vi "Motor with Encoder - DrH Test v2.vi"() -> ()   [LabVIEW 2016]
doc: "This example shows how to move a motor connected to an encoder and a wheel, and then read information about the system from an encoder.\n\nThis is an example of how to use feedback (from the encoder) to create an open loop system. If some control method was used, for example using PID, a closed loop system could be created.\n\nThis example expects a USB cable connected from your development PC to the Type B USB Jack (next to the power input) on the roboRIO.\n\nThis example requires the Driver Station to be running with Teleoperated Enabled."
uses:
  <vilib>/Rock Robotics/SystemInterfaces/DIO/FPGA_DIOChannel.ctl
  <vilib>/Rock Robotics/WPI/Encoder/WPI_EncoderType.ctl
  <vilib>/Rock Robotics/SystemInterfaces/DIO/FPGA_DIOPWMChannel.ctl
  <vilib>/Rock Robotics/WPI/Counter/WPI_CounterDigitalInputToDigitalSource.vi
  <vilib>/Rock Robotics/WPI/MotorControl/WPI_MotorControlOpen SPARK.vi
panel:
  out "Encoder Rate (RPM) 2":dbl
  out "XY Graph":cluster{dbl[], dbl[]}(graph)
  out "Waveform Chart":dbl(graph)
  in  "Motor Speed (-1 to 1)":dbl(slide) scale=-1.0..1.0
  in  "Motor PWM Channel":T1=enum."PWM 9"
  in  "Number Samples to Average":u8=1 min=1 max=128
  in  "Invert Direction":bool
  in  "Decoding Type":T2=enum."4x"
  in  "DistancePerCount (deg)":dbl=0.351563
  in  "Encoder B Channel":T3=enum."DIO 1"
  in  "Encoder A Channel":T3
  out "Encoder Rate (deg/sec)":dbl
  in  "Minimum Rate":dbl=20.0
  in  "Stop":bool
  out "Encoder Alarm Status":string="Encoder Stopped"
  out "Encoder Direction":string="Forward"
  # "These can be set while running."
  # "Output information."
  # "Set these inputs before running."
  # "This example requires the Driver Station to be running with Teleoperated Enabled."
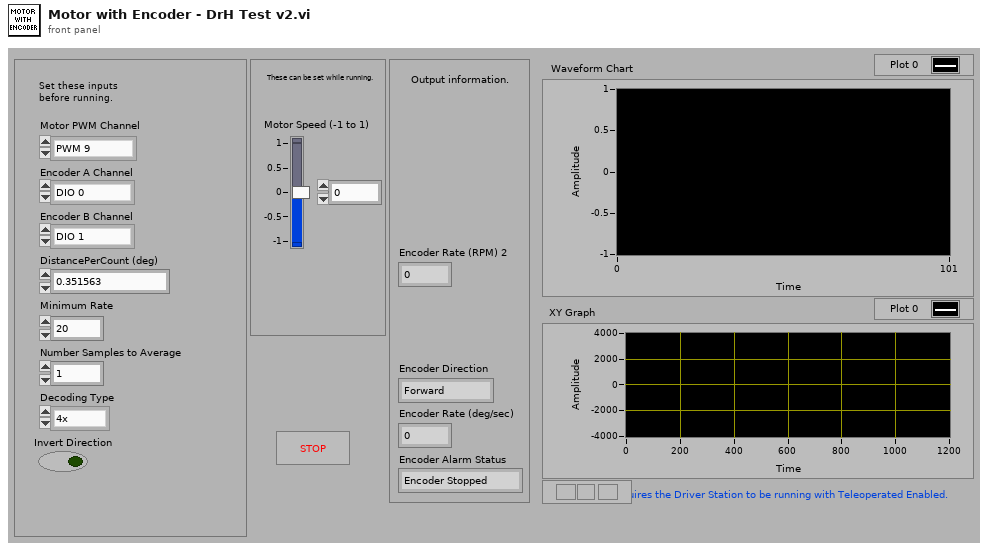
[diagram p1: front panel]
types:
  T1 = typedef "FPGA_DIOPWMChannel.ctl" = enum8{"PWM 0", "PWM 1", "PWM 2", "PWM 3", "PWM 4", "PWM 5", "PWM 6", "PWM 7", "PWM 8", "PWM 9", "PWM MXP 0", "PWM MXP 1", "PWM MXP 2", "PWM MXP 3", "PWM MXP 4", "PWM MXP 5", "PWM MXP 6", "PWM MXP 7", "PWM MXP 8", "PWM MXP 9", "Invalid"}
  T2 = typedef "WPI_EncoderType.ctl" = enum16{"1x", "2x", "4x"}
  T3 = typedef "FPGA_DIOChannel.ctl" = enum8{"DIO 0", "DIO 1", "DIO 2", "DIO 3", "DIO 4", "DIO 5", "DIO 6", "DIO 7", "DIO 8", "DIO 9", "DIO MXP 0", "DIO MXP 1", "DIO MXP 2", "DIO MXP 3", "DIO MXP 4", "DIO MXP 5", "DIO MXP 6", "DIO MXP 7", "DIO MXP 8", "DIO MXP 9", "DIO MXP 10", "DIO MXP 11", "DIO MXP 12", "DIO MXP 13", "DIO MXP 14", "DIO MXP 15", "SPI Port CS1", "SPI Port CS2", "SPI Port CS3", "SPI Port MISO", "SPI Port MOSI", "Invalid"}
  T4 = typedef "WPI_MotorControlDeviceRef.ctl" = cluster{"DeviceStatus":errorcluster, "Type":T5, "PWM":cluster{"PWM Channel":T1, "DeadBand":T6}, "CAN":cluster{"Device Number":u8, "SetOutput VI Ref":variant, "GetOutput VI Ref":variant, "Enable VI Ref":variant, "Disable VI Ref":variant, "Data":variant}, "Invert":bool}
  T5 = typedef "WPI_MotorControlType.ctl" = enum16{"PWM", "CAN"}
  T6 = typedef "WPI_PWMDeadband.ctl" = cluster{"Name":string, "maxPositivePwm":i32, "minPositivePwm":i32, "centerPwm":i32, "maxNegativePwm":i32, "minNegativePwm":i32, "angularRange":u16}
  T7 = typedef "WPI_DigitalInputDevRef.ctl" = cluster{"DevStatus":errorcluster, "DIO Channel":T3}
  T8 = typedef "FPGA_CounterEncoderSourceConvertionLVSourceType.ctl" = cluster{"DevStatus":errorcluster, "AnalogTriggerMode?":bool, "DigitalMode":cluster{"DIO Channel":T9}, "AnalogTriggerMode":cluster{"AnalogTriggerIndex":T10, "OutputType":T11}}
  T9 = typedef "FPGA_DIODigitalSourceChannel.ctl" = enum8{"DIO 0", "DIO 1", "DIO 2", "DIO 3", "DIO 4", "DIO 5", "DIO 6", "DIO 7", "DIO 8", "DIO 9", "DIO MXP 0", "DIO MXP 1", "DIO MXP 2", "DIO MXP 3", "DIO MXP 4", "DIO MXP 5", "DIO MXP 6", "DIO MXP 7", "DIO MXP 8", "DIO MXP 9", "DIO MXP 10", "DIO MXP 11", "DIO MXP 12", "DIO MXP 13", "DIO MXP 14", "DIO MXP 15", "Disabled"}
  T10 = typedef "FPGA_AnalogTriggerIndex.ctl" = enum8{"Trig 0", "Trig 1", "Trig 2", "Trig 3", "Trig 4", "Trig 5", "Trig 6", "Trig 7", "Invalid"}
  T11 = typedef "FPGA_AnalogTriggerOutType.ctl" = enum16{"InWindow", "TriggerState", "Rising", "Falling"}
  T12 = typedef "WPI_EncoderDevRef.ctl" = cluster{"DevStatus":errorcluster, "EncoderIndex":T13, "CounterIndex":T14, "DistancePerCount":dbl, "Decoding Type":T2}
  T13 = typedef "FPGA_EncoderIdx.ctl" = enum8{"Enc 0", "Enc 1", "Enc 2", "Enc 3", "Enc 4", "Enc 5", "Enc 6", "Enc 7", "Invalid"}
  T14 = typedef "FPGA_CounterCtrSystemIndex.ctl" = enum8{"Ctr 0", "Ctr 1", "Ctr 2", "Ctr 3", "Ctr 4", "Ctr 5", "Ctr 6", "Ctr 7", "Invalid"}
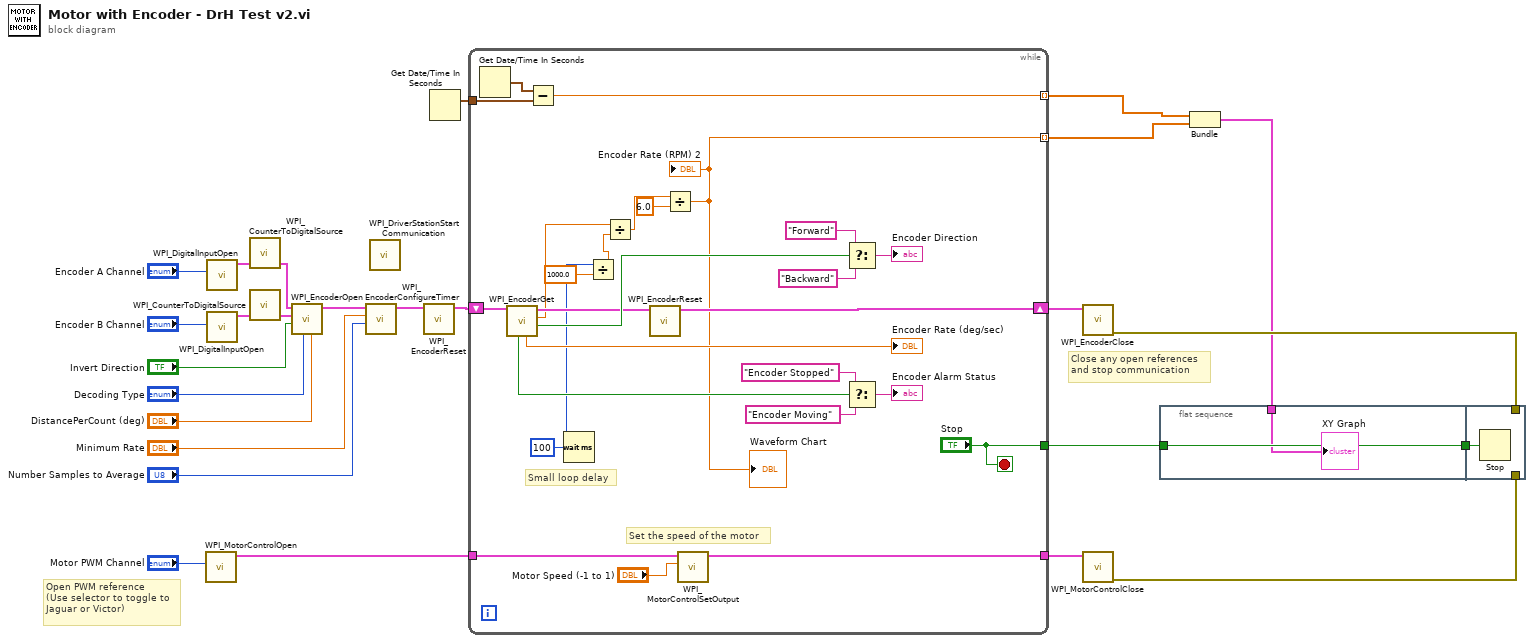
[diagram p0: block diagram]
diagram:
  # "Open PWM reference\n(Use selector to toggle to Jaguar or Victor)"
  # "Close any open references\nand stop communication"
  n1 = call-poly <vilib>:"WPI_MotorControlOpen.vi"("PWM Channel"="Motor PWM Channel") -> ("MotorControlDeviceRef"=w12:T4)  [unwired: 3 in, 7 out]
  n2 = call <vilib>:"WPI_DigitalInputOpen.vi"("DIO Channel"="Encoder A Channel") -> ("DigitalInputDevRef"=w23:T7)  [unwired: 1 in, 9 out]
  n3 = call <vilib>:"WPI_DigitalInputOpen.vi"("DIO Channel"="Encoder B Channel") -> ("DigitalInputDevRef"=w24:T7)  [unwired: 1 in, 9 out]
  n4 = call-poly <vilib>:"WPI_CounterToDigitalSource.vi"("DigitalInputDevRef"=w23) -> ("Digital Source"=w22:T8)  [unwired: 6 out]
  n5 = call-poly <vilib>:"WPI_CounterToDigitalSource.vi"("DigitalInputDevRef"=w24) -> ("Digital Source"=w25:T8)  [unwired: 6 out]
  n6 = call <vilib>:"WPI_EncoderOpen.vi"("DistancePerCount"="DistancePerCount (deg)", "Decoding Type"="Decoding Type", "Invert Direction (False)"="Invert Direction", "BSource"=w25, "ASource"=w22) -> ("EncoderDevRef"=w16:T12)  [unwired: 3 in, 3 out]
  n7 = call <vilib>:"WPI_EncoderConfigureTimer.vi"("Number Samples to Average"="Number Samples to Average", "Minimum Rate"="Minimum Rate", "EncoderDevRef"=w16) -> ("EncoderDevRef"=w4:T12)  [unwired: 1 in, 7 out]
  n8 = call <vilib>:"WPI_DriverStationStart Communication.vi"() -> ()  [unwired: 2 in, 10 out]
  n9 = call <vilib>:"WPI_EncoderReset.vi"("EncoderDevRef"=w4) -> ("EncoderDevRef"=w3:T12)  [unwired: 1 in, 9 out]
  n10 = Get Date/Time In Seconds() -> (seconds since 1Jan1904=w7:timestamp)
  n11 = while {
    shift-right: [w34] -> w26
    shift-left: w3 -> [w36]
    tunnel: ["Stop"] -> w10
    tunnel: w12 -> [w44]
    tunnel: [w43] -> w13
    tunnel: [w27] -> w5 mode=indexing
    tunnel: w7 -> [w39]
    tunnel: [w38] -> w6 mode=indexing
    stop <- "Stop" stop-if-true
    w31 = u32 100 ("milliseconds to wait")
    # "Set the speed of the motor"
    # "Small loop delay"
    n12 = Get Date/Time In Seconds() -> (seconds since 1Jan1904=w40:timestamp)
    n13 = call <vilib>:"WPI_EncoderGet.vi"("EncoderDevRef"=w36) -> ("Direction"=w50:bool, "Distance"=w33:dbl, "EncoderDevRef"=w35:T12, "Rate"=→"Encoder Rate (deg/sec)":dbl, "Stopped"=w49:bool)  [unwired: 1 in, 5 out]
    n14 = Subtract(x=w40, y=w39) -> (x-y=w38:dbl)
    n15 = Wait (ms)(milliseconds to wait=w31) -> ()  [unwired: 1 out]
    n16 = Divide(x=w31, y=1000.0) -> (x/y=w30:dbl)
    n17 = Divide(x=w33, y=w30) -> (x/y=w28:dbl)
    n18 = call <vilib>:"WPI_EncoderReset.vi"("EncoderDevRef"=w35) -> ("EncoderDevRef"=w34:T12)  [unwired: 1 in, 9 out]
    n19 = Divide(x=w28, y=6.0) -> (x/y=w27:dbl)
    "Waveform Chart" <- w27
    "Encoder Rate (RPM) 2" <- w27
    n20 = call <vilib>:"WPI_MotorControlSetOutput.vi"("Output"="Motor Speed (-1 to 1)", "MotorControlDevRef"=w44) -> ("MotorControlDevRef"=w43:T4)  [unwired: 2 in, 7 out]
    n21 = Select(t="Forward", s=w50, f="Backward") -> (s? t:f=→"Encoder Direction":string)
    n22 = Select(t="Encoder Stopped", s=w49, f="Encoder Moving") -> (s? t:f=→"Encoder Alarm Status":string)
  }
  n23 = call <vilib>:"WPI_EncoderClose.vi"("EncoderDevRef"=w26) -> ("error out"=w9:errorcluster)  [unwired: 2 in, 8 out]
  n24 = call <vilib>:"WPI_MotorControlClose.vi"("MotorControlDevRef"=w13) -> ("error out"=w8:errorcluster)  [unwired: 1 in, 9 out]
  n25 = flat-sequence {
    tunnel: w10 -> [w54]
    tunnel: [w54] -> w2
    tunnel: w1 -> [w53]
    tunnel: w9 -> [_]
    tunnel: w8 -> [_]
    tunnel: w2 -> [w55]
    frame #0 {
      "XY Graph" <- w53
    }
    frame #1 {
      n26 = Stop(stop? (T)=w55) -> ()
    }
  }
  n27 = Bundle(w6, w5) -> (w1:cluster{dbl[], dbl[]})  [unwired: 1 in]
